vi "LSMcontroller_v64_updatedwaveformhandling.vi"() -> ()   [LabVIEW 2015] (continued)
                n4212 = call "waveformsAObuffer.vi"("command"="get") -> ("AO wf out"=w1168:waveform(dbl)[])  [unwired: 1 in]
                n4213 = local read "wavdet"() -> (w1158:bool)
                n4214 = call "waveformsDObuffer.vi"("command"="get") -> ("DO wf out"=w1164:digitalwaveform[])  [unwired: 1 in]
                n4215 = call "correctwaveformsizetemp.vi"("new sampling frequency (Hz)"=w1155, "start"=FALSE, "reference waveforms to"=w1159, "Analog waveforms in"=w1168, "stop"=FALSE, "Digital waveforms in"=w1164) -> ("analog wf out"=w1162:waveform(dbl)[], "Digital wf out"=w1160:digitalwaveform[], "measpoints"=w1157:i32)
                n4216 = local write "Analog Lines Plot"(w1162) -> ()
                n4217 = call "GetNumCamFramesv2.vi"("Digital Waveform Graph"=w1160) -> ("Numeric"=w1161:i32)  [unwired: 10 in]
                n4218 = local write "Digital Lines Plot"(w1160) -> ()
                n4219 = call "waveformsDObuffer.vi"("DO wf in"=w1160, "command"="set") -> ()  [unwired: 1 out]
                n4220 = call "waveformsAObuffer.vi"("AO wf in"=w1162, "command"="set") -> ()  [unwired: 1 out]
                n4221 = local write "Total Camera Frames"(w1161) -> ()
                n4222 = case shown="True" w1158 {
                  tunnel: w1157 -> [_ w1171]
                  frame False {
                  }
                  frame True {
                    n4223 = local write "# of frames"(w1171) -> ()
                  }
                }
              }
              frame #3 {
                n4224 = local read "finite samples"() -> (w1172:bool)
                n4225 = local read "continuous"() -> (w1173:bool)
                n4226 = local read "wavdet"() -> (w1174:bool)
                n4227 = call "2pparameters.vi"("command"="get") -> ("params out"=w1177:T10)  [unwired: 1 in]
                n4228 = Bundle By Name(cluster=w1177, "finite"=w1172, "cont"=w1173, "wavdet"=w1174) -> (w1175:T10)
                n4229 = call "2pparameters.vi"("Params in"=w1175, "command"="set") -> ()  [unwired: 1 out]
              }
            }
          }
          event "load changed AOsq": Value Change {
            n4230 = event-data() -> ("NewVal"=w1179:bool)  [unwired: 1 in, 5 out]
            n4231 = case shown="True" w1179 {
              frame False {
              }
              frame True {
                n4232 = stacked-sequence {
                  seq-local: [_ _ w1287 _ _] -> [_ _ _ w1309 _]
                  seq-local: [_ _ w1286 _ _] -> [_ _ _ w1308 _]
                  frame #0 {
                    n4233 = local read "Measurement"() -> (w1181:T4)
                    n4234 = local write "changeAOsq"(TRUE ("addAO")) -> ()
                    n4235 = case shown="\"X-Y-t movie\", Default" w1181 {
                      frame "X-Y-t movie", Default {
                        n4236 = local read "avpp"() -> (w1202:i32)
                        n4237 = local read "Angle ref"() -> (w1201:dbl)
                        n4238 = local read "ROI Type"() -> (w1200:u16)
                        n4239 = local read "xpixels ref"() -> (w1197:i32)
                        n4240 = local read "Vx-min ref"() -> (w1196:dbl)
                        n4241 = local read "Vx-max ref"() -> (w1195:dbl)
                        n4242 = local read "ypixels ref"() -> (w1193:i32)
                        n4243 = local read "Vy-min ref"() -> (w1194:dbl)
                        n4244 = local read "Vy-max ref"() -> (w1190:dbl)
                        n4245 = local read "Sampling rate"() -> (w1184:dbl)
                        n4246 = local read "finite samples"() -> (w1185:bool)
                        n4247 = local read "continuous"() -> (w1188:bool)
                        n4248 = local read "wavdet"() -> (w1189:bool)
                        n4249 = local read "# of frames"() -> (w1187:i32)
                        n4250 = local read "maxbufferAI"() -> (w1186:i32)
                        n4251 = local read "Override AI buffer"() -> (w1182:bool)
                        n4252 = call "2pparameters.vi"("command"="get") -> ("params out"=w1199:T10)  [unwired: 1 in]
                        n4253 = Bundle By Name(cluster=w1199, "type"="X-Y-t movie", "avpp"=w1202, "Angle Img"=w1201, "Xpixels Img"=w1197, "Vx-min Img"=w1196, "VX-max Img"=w1195, "Ypixels Img"=w1193, "Vy-min Img"=w1194, "Vy-max Img"=w1190, "srate"=w1184, "srate Img"=w1184, "finite"=w1185, "cont"=w1188, "wavdet"=w1189, "measpoints"=w1187, "maxbufferAI"=w1186, "Drawing Mode"=w1200, "Vz-reset"=0.0, "AIoverride"=w1182) -> (w1191:T10)
                        n4254 = call "2pparameters.vi"("Params in"=w1191, "command"="set") -> ()  [unwired: 1 out]
                      }
                      frame "X-Y-Z stack" {
                        n4255 = call "2pparameters.vi"("command"="get") -> ("params out"=w1206:T10)  [unwired: 1 in]
                        n4256 = Bundle By Name(cluster=w1206, "type"="X-Y-Z stack") -> (w1204:T10)
                        n4257 = call "2pparameters.vi"("Params in"=w1204, "command"="set") -> ()  [unwired: 1 out]
                      }
                      frame "Lifetime (scan)" {
                        n4258 = call "2pparameters.vi"("command"="get") -> ("params out"=w1211:T10)  [unwired: 1 in]
                        n4259 = Bundle By Name(cluster=w1211, "type"="Lifetime (scan)") -> (w1209:T10)
                        n4260 = call "2pparameters.vi"("Params in"=w1209, "command"="set") -> ()  [unwired: 1 out]
                      }
                      frame "Lifetime (contour)" {
                        n4261 = local read "Vy-min draw"() -> (w1221:dbl)
                        n4262 = local read "Vy-max draw"() -> (w1220:dbl)
                        n4263 = local read "Vx-min draw"() -> (w1223:dbl)
                        n4264 = local read "Vx-max draw"() -> (w1222:dbl)
                        n4265 = local read "xpixels ref"() -> (w1219:i32)
                        n4266 = local read "ypixels ref"() -> (w1218:i32)
                        n4267 = local read "ROI Type"() -> (w1217:u16)
                        n4268 = local read "srateAODOtt"() -> (w1228:dbl)
                        n4269 = local read "# of frames"() -> (w1233:i32)
                        n4270 = local read "refreshtime"() -> (w1225:dbl)
                        n4271 = local read "Pel"() -> (w1216:dbl)
                        n4272 = local read "bin"() -> (w1231:dbl)
                        n4273 = local read "Override AI buffer"() -> (w1214:bool)
                        n4274 = local read "finite samples"() -> (w1240:bool)
                        n4275 = local read "srateAODOtt"() -> (w1227:dbl)
                        n4276 = local read "srateAODOtt"() -> (w1234:dbl)
                        n4277 = local read "continuous"() -> (w1239:bool)
                        n4278 = local read "Angle ref"() -> (w1224:dbl)
                        n4279 = local read "wavdet"() -> (w1241:bool)
                        n4280 = local read "Vx-ref"() -> (w1236:dbl)
                        n4281 = local read "Vy-ref"() -> (w1238:dbl)
                        n4282 = local read "avpp"() -> (w1237:i32)
                        n4283 = call "tt_timeandsamples.vi"("bin"=w1231, "refreshtime"=w1225, "srateAODOtt"=w1228, "tot#ofsamples"=w1233) -> ("refreshrate"=w1229:dbl, "refreshbuffer"=w1230:i32, "timetracecycles"=w1235:i32)  [unwired: 5 in]
                        n4284 = local read "bin"() -> (w1232:dbl)
                        n4285 = call "2pparameters.vi"("command"="get") -> ("params out"=w1244:T10)  [unwired: 1 in]
                        n4286 = Bundle By Name(cluster=w1244, "Drawing Mode"=w1217, "measpoints"=w1233, "tt_cycles"=w1235, "refreshbuffer"=w1230, "refreshrate"=w1229, "Vx-ref"=w1236, "Vy-ref"=w1238, "srate"=w1227, "finite"=w1240, "cont"=w1239, "wavdet"=w1241, "avpp"=w1237, "srateAODO"=w1234, "bufferAI"=w1230, "bin"=w1232, "Angle Img"=w1224, "Vxminref"=w1223, "Vxmaxref"=w1222, "Vyminref"=w1221, "Vymaxref"=w1220, "Xpixels Img"=w1219, "Ypixels Img"=w1218, "Pel"=w1216, "Vz-reset"=0.0, "AIoverride"=w1214, "type"="Lifetime (contour)") -> (w1242:T10)
                        n4287 = Reciprocal(x=w1229) -> (1/x=w1226:dbl)
                        n4288 = local write "refreshtime"(w1226) -> ()
                        n4289 = call "2pparameters.vi"("Params in"=w1242, "command"="set") -> ()  [unwired: 1 out]
                      }
                      frame "X-Y-Z-t movie" {
                      }
                      frame "linescan" {
                      }
                      frame "Timetrace" {
                        n4290 = local read "Vy-min draw"() -> (w1254:dbl)
                        n4291 = local read "Vy-max draw"() -> (w1253:dbl)
                        n4292 = local read "Vx-min draw"() -> (w1256:dbl)
                        n4293 = local read "Vx-max draw"() -> (w1255:dbl)
                        n4294 = local read "xpixels ref"() -> (w1252:i32)
                        n4295 = local read "ypixels ref"() -> (w1251:i32)
                        n4296 = local read "ROI Type"() -> (w1250:u16)
                        n4297 = local read "srateAODOtt"() -> (w1261:dbl)
                        n4298 = local read "# of frames"() -> (w1266:i32)
                        n4299 = local read "refreshtime"() -> (w1258:dbl)
                        n4300 = local read "Pel"() -> (w1249:dbl)
                        n4301 = local read "bin"() -> (w1264:dbl)
                        n4302 = local read "Override AI buffer"() -> (w1247:bool)
                        n4303 = local read "finite samples"() -> (w1273:bool)
                        n4304 = local read "srateAODOtt"() -> (w1260:dbl)
                        n4305 = local read "srateAODOtt"() -> (w1267:dbl)
                        n4306 = local read "continuous"() -> (w1272:bool)
                        n4307 = local read "Angle ref"() -> (w1257:dbl)
                        n4308 = local read "wavdet"() -> (w1274:bool)
                        n4309 = local read "Vx-ref"() -> (w1269:dbl)
                        n4310 = local read "Vy-ref"() -> (w1271:dbl)
                        n4311 = local read "avpp"() -> (w1270:i32)
                        n4312 = call "tt_timeandsamples.vi"("bin"=w1264, "refreshtime"=w1258, "srateAODOtt"=w1261, "tot#ofsamples"=w1266) -> ("refreshrate"=w1262:dbl, "refreshbuffer"=w1263:i32, "timetracecycles"=w1268:i32)  [unwired: 5 in]
                        n4313 = local read "bin"() -> (w1265:dbl)
                        n4314 = call "2pparameters.vi"("command"="get") -> ("params out"=w1277:T10)  [unwired: 1 in]
                        n4315 = Bundle By Name(cluster=w1277, "Drawing Mode"=w1250, "measpoints"=w1266, "tt_cycles"=w1268, "refreshbuffer"=w1263, "refreshrate"=w1262, "Vx-ref"=w1269, "Vy-ref"=w1271, "srate"=w1260, "finite"=w1273, "cont"=w1272, "wavdet"=w1274, "avpp"=w1270, "srateAODO"=w1267, "bufferAI"=w1263, "bin"=w1265, "Angle Img"=w1257, "Vxminref"=w1256, "Vxmaxref"=w1255, "Vyminref"=w1254, "Vymaxref"=w1253, "Xpixels Img"=w1252, "Ypixels Img"=w1251, "Pel"=w1249, "Vz-reset"=0.0, "AIoverride"=w1247, "type"="Timetrace") -> (w1275:T10)
                        n4316 = Reciprocal(x=w1262) -> (1/x=w1259:dbl)
                        n4317 = local write "refreshtime"(w1259) -> ()
                        n4318 = call "2pparameters.vi"("Params in"=w1275, "command"="set") -> ()  [unwired: 1 out]
                      }
                      frame "Lifetime (point)" {
                      }
                    }
                  }
                  frame #1 {
                    w1280 = FALSE ("wavdet")
                    n4319 = call "2pparameters.vi"("command"="get") -> ("params out"=w1284:T10)  [unwired: 1 in]
                    n4320 = Bundle By Name(cluster=w1284, "finite"=w1280, "cont"=w1280, "wavdet"=TRUE) -> (w1281:T10)
                    n4321 = call "2pparameters.vi"("Params in"=w1281, "command"="set") -> ()  [unwired: 1 out]
                  }
                  frame #2 {
                    n4322 = local read "AO channels"() -> (w1289:u32)
                    n4323 = call "2pparameters.vi"("command"="get") -> ("params out"=w1291:T10)  [unwired: 1 in]
                    n4324 = Unbundle By Name(w1291) -> ("aAO"=w1290:u32[])
                    n4325 = Search 1D Array(1D array=w1290, element=w1289) -> (index of element=w1287:i32)  [unwired: 1 in]
                    n4326 = Greater?(x=w1287, y=-1) -> (0:w1286:bool)
                    n4327 = case shown="True" w1286 {
                      tunnel: w1287 -> [_ w1305]
                      frame False {
                      }
                      frame True {
                        n4328 = local read "Meastab"() -> (w1294:enum32{"X-Y Image", "Linescan", "Timetrace"})
                        n4329 = case shown="\"Timetrace\"" w1294 {
                          tunnel: [w1306 w1307] -> w1293
                          frame "X-Y Image", Default {
                            n4330 = local read "Sampling rate"() -> (w1306:dbl)
                          }
                          frame "Timetrace" {
                            n4331 = local read "srateAODOtt"() -> (w1307:dbl)
                          }
                        }
                        n4332 = local read "Start amplitude (V)"() -> (w1302:dbl)
                        n4333 = local read "phase shift (ms)"() -> (w1297:dbl)
                        n4334 = local read "Step size (V)"() -> (w1300:dbl)
                        n4335 = local read "Baseline (V)"() -> (w1301:dbl)
                        n4336 = local read "Period (ms)"() -> (w1298:dbl)
                        n4337 = local read "padding value"() -> (w1295:dbl)
                        n4338 = local read "Repeats"() -> (w1304:dbl)
                        n4339 = local read "Cycles"() -> (w1303:dbl)
                        n4340 = local read "DC (%)"() -> (w1299:dbl)
                        n4341 = local read "Pulses"() -> (w1296:dbl)
                        n4342 = call "replace AO square wf param.vi"("Baseline (V)"=w1301, "Start amplitude (V)"=w1302, "Cycles"=w1303, "Repeats"=w1304, "index of AO wave"=w1305, "Step size (V)"=w1300, "DC (%)"=w1299, "Sampling frequency (Hz)"=w1293, "Period (ms)"=w1298, "Cycle length (s)"=w1297, "Pulses"=w1296, "padding value"=w1295) -> ()  [unwired: 4 in]
                      }
                    }
                  }
                  frame #3 {
                    n4343 = case shown="True" w1308 {
                      tunnel: w1309 -> [_ w1317]
                      frame False {
                      }
                      frame True {
                        n4344 = call "waveformparamsv2.vi"("command"="get") -> ("Params out"=w1331:T14)  [unwired: 4 in, 2 out]
                        n4345 = Unbundle By Name(w1331) -> ("AO parameters"=w1330:T15)
                        n4346 = local read "Meastab"() -> (w1312:enum32{"X-Y Image", "Linescan", "Timetrace"})
                        n4347 = case shown="\"Timetrace\"" w1312 {
                          tunnel: [w1333 w1334] -> w1321
                          frame "X-Y Image", Default {
                            n4348 = local read "Sampling rate"() -> (w1333:dbl)
                          }
                          frame "Timetrace" {
                            n4349 = local read "srateAODOtt"() -> (w1334:dbl)
                          }
                        }
                        n4350 = Index Array(array=w1330, index=w1317) -> (element=w1319:T16)
                        n4351 = call "waveformsAObuffer.vi"("command"="get") -> ("AO wf out"=w1318:waveform(dbl)[])  [unwired: 1 in]
                        n4352 = call "generateRampedSquareWave_fromAOparameters.vi"("AO params"=w1319) -> ("Waveform"=w1316:waveform(dbl))  [unwired: 1 out]
                        n4353 = property on="refwf" class="Ring (strict)"() -> ("RingText.Text"=w1320:string)  [unwired: 2 in, 2 out]
                        n4354 = Replace Array Subset(array=w1318, new element=w1316, index=w1317) -> (w1315:waveform(dbl)[])
                        n4355 = call "waveformsDObuffer.vi"("command"="get") -> ("DO wf out"=w1326:digitalwaveform[])  [unwired: 1 in]
                        n4356 = call "correctwaveformsizetemp.vi"("new sampling frequency (Hz)"=w1321, "start"=FALSE, "reference waveforms to"=w1320, "Analog waveforms in"=w1315, "stop"=FALSE, "Digital waveforms in"=w1326) -> ("analog wf out"=w1324:waveform(dbl)[], "Digital wf out"=w1322:digitalwaveform[], "measpoints"=w1313:i32)
                        n4357 = local read "wavdet"() -> (w1314:bool)
                        n4358 = local write "Analog Lines Plot"(w1324) -> ()
                        n4359 = call "GetNumCamFramesv2.vi"("Digital Waveform Graph"=w1322) -> ("Numeric"=w1323:i32)  [unwired: 10 in]
                        n4360 = local write "Digital Lines Plot"(w1322) -> ()
                        n4361 = call "waveformsAObuffer.vi"("AO wf in"=w1324, "command"="set") -> ()  [unwired: 1 out]
                        n4362 = call "waveformsDObuffer.vi"("DO wf in"=w1322, "command"="set") -> ()  [unwired: 1 out]
                        n4363 = local write "Total Camera Frames"(w1323) -> ()
                        n4364 = case shown="True" w1314 {
                          tunnel: w1313 -> [_ w1335]
                          frame False {
                          }
                          frame True {
                            n4365 = local write "# of frames"(w1335) -> ()
                          }
                        }
                      }
                    }
                  }
                  frame #4 {
                    w1337 = FALSE ("addAO")
                    n4366 = local read "finite samples"() -> (w1338:bool)
                    n4367 = local read "continuous"() -> (w1339:bool)
                    n4368 = local read "wavdet"() -> (w1340:bool)
                    n4369 = local write "changeAOsq"(w1337) -> ()
                    n4370 = property on="load changed AOsq" class="Bool (strict)"("Val(Sgnl)"=w1337) -> ()  [unwired: 2 in, 2 out]
                    n4371 = call "2pparameters.vi"("command"="get") -> ("params out"=w1343:T10)  [unwired: 1 in]
                    n4372 = Bundle By Name(cluster=w1343, "finite"=w1338, "cont"=w1339, "wavdet"=w1340) -> (w1341:T10)
                    n4373 = local write "not loaded"(FALSE ("not loaded")) -> ()
                    n4374 = call "2pparameters.vi"("Params in"=w1341, "command"="set") -> ()  [unwired: 1 out]
                  }
                }
              }
            }
          }
          event "load changed AOtri": Value Change {
            n4375 = event-data() -> ("NewVal"=w1345:bool)  [unwired: 1 in, 5 out]
            n4376 = case shown="True" w1345 {
              frame False {
              }
              frame True {
                n4377 = stacked-sequence {
                  seq-local: [_ _ w1453 _ _] -> [_ _ _ w1471 _]
                  seq-local: [_ _ w1452 _ _] -> [_ _ _ w1470 _]
                  frame #0 {
                    n4378 = local read "Measurement"() -> (w1347:T4)
                    n4379 = local write "changeAOtri"(TRUE ("addAO")) -> ()
                    n4380 = case shown="\"X-Y-t movie\", Default" w1347 {
                      frame "X-Y-t movie", Default {
                        n4381 = local read "avpp"() -> (w1368:i32)
                        n4382 = local read "Angle ref"() -> (w1367:dbl)
                        n4383 = local read "ROI Type"() -> (w1366:u16)
                        n4384 = local read "xpixels ref"() -> (w1363:i32)
                        n4385 = local read "Vx-min ref"() -> (w1362:dbl)
                        n4386 = local read "Vx-max ref"() -> (w1361:dbl)
                        n4387 = local read "ypixels ref"() -> (w1359:i32)
                        n4388 = local read "Vy-min ref"() -> (w1360:dbl)
                        n4389 = local read "Vy-max ref"() -> (w1356:dbl)
                        n4390 = local read "Sampling rate"() -> (w1350:dbl)
                        n4391 = local read "finite samples"() -> (w1351:bool)
                        n4392 = local read "continuous"() -> (w1354:bool)
                        n4393 = local read "wavdet"() -> (w1355:bool)
                        n4394 = local read "# of frames"() -> (w1353:i32)
                        n4395 = local read "maxbufferAI"() -> (w1352:i32)
                        n4396 = local read "Override AI buffer"() -> (w1348:bool)
                        n4397 = call "2pparameters.vi"("command"="get") -> ("params out"=w1365:T10)  [unwired: 1 in]
                        n4398 = Bundle By Name(cluster=w1365, "type"="X-Y-t movie", "avpp"=w1368, "Angle Img"=w1367, "Xpixels Img"=w1363, "Vx-min Img"=w1362, "VX-max Img"=w1361, "Ypixels Img"=w1359, "Vy-min Img"=w1360, "Vy-max Img"=w1356, "srate"=w1350, "srate Img"=w1350, "finite"=w1351, "cont"=w1354, "wavdet"=w1355, "measpoints"=w1353, "maxbufferAI"=w1352, "Drawing Mode"=w1366, "Vz-reset"=0.0, "AIoverride"=w1348) -> (w1357:T10)
                        n4399 = call "2pparameters.vi"("Params in"=w1357, "command"="set") -> ()  [unwired: 1 out]
                      }
                      frame "X-Y-Z stack" {
                        n4400 = call "2pparameters.vi"("command"="get") -> ("params out"=w1372:T10)  [unwired: 1 in]
                        n4401 = Bundle By Name(cluster=w1372, "type"="X-Y-Z stack") -> (w1370:T10)
                        n4402 = call "2pparameters.vi"("Params in"=w1370, "command"="set") -> ()  [unwired: 1 out]
                      }
                      frame "Lifetime (scan)" {
                        n4403 = call "2pparameters.vi"("command"="get") -> ("params out"=w1377:T10)  [unwired: 1 in]
                        n4404 = Bundle By Name(cluster=w1377, "type"="Lifetime (scan)") -> (w1375:T10)
                        n4405 = call "2pparameters.vi"("Params in"=w1375, "command"="set") -> ()  [unwired: 1 out]
                      }
                      frame "Lifetime (contour)" {
                        n4406 = local read "Vy-min draw"() -> (w1387:dbl)
                        n4407 = local read "Vy-max draw"() -> (w1386:dbl)
                        n4408 = local read "Vx-min draw"() -> (w1389:dbl)
                        n4409 = local read "Vx-max draw"() -> (w1388:dbl)
                        n4410 = local read "xpixels ref"() -> (w1385:i32)
                        n4411 = local read "ypixels ref"() -> (w1384:i32)
                        n4412 = local read "ROI Type"() -> (w1383:u16)
                        n4413 = local read "srateAODOtt"() -> (w1394:dbl)
                        n4414 = local read "# of frames"() -> (w1399:i32)
                        n4415 = local read "refreshtime"() -> (w1391:dbl)
                        n4416 = local read "Pel"() -> (w1382:dbl)
                        n4417 = local read "bin"() -> (w1397:dbl)
                        n4418 = local read "Override AI buffer"() -> (w1380:bool)
                        n4419 = local read "finite samples"() -> (w1406:bool)
                        n4420 = local read "srateAODOtt"() -> (w1393:dbl)
                        n4421 = local read "srateAODOtt"() -> (w1400:dbl)
                        n4422 = local read "continuous"() -> (w1405:bool)
                        n4423 = local read "Angle ref"() -> (w1390:dbl)
                        n4424 = local read "wavdet"() -> (w1407:bool)
                        n4425 = local read "Vx-ref"() -> (w1402:dbl)
                        n4426 = local read "Vy-ref"() -> (w1404:dbl)
                        n4427 = local read "avpp"() -> (w1403:i32)
                        n4428 = call "tt_timeandsamples.vi"("bin"=w1397, "refreshtime"=w1391, "srateAODOtt"=w1394, "tot#ofsamples"=w1399) -> ("refreshrate"=w1395:dbl, "refreshbuffer"=w1396:i32, "timetracecycles"=w1401:i32)  [unwired: 5 in]
                        n4429 = local read "bin"() -> (w1398:dbl)
                        n4430 = call "2pparameters.vi"("command"="get") -> ("params out"=w1410:T10)  [unwired: 1 in]
                        n4431 = Bundle By Name(cluster=w1410, "Drawing Mode"=w1383, "measpoints"=w1399, "tt_cycles"=w1401, "refreshbuffer"=w1396, "refreshrate"=w1395, "Vx-ref"=w1402, "Vy-ref"=w1404, "srate"=w1393, "finite"=w1406, "cont"=w1405, "wavdet"=w1407, "avpp"=w1403, "srateAODO"=w1400, "bufferAI"=w1396, "bin"=w1398, "Angle Img"=w1390, "Vxminref"=w1389, "Vxmaxref"=w1388, "Vyminref"=w1387, "Vymaxref"=w1386, "Xpixels Img"=w1385, "Ypixels Img"=w1384, "Pel"=w1382, "Vz-reset"=0.0, "AIoverride"=w1380, "type"="Lifetime (contour)") -> (w1408:T10)
                        n4432 = Reciprocal(x=w1395) -> (1/x=w1392:dbl)
                        n4433 = local write "refreshtime"(w1392) -> ()
                        n4434 = call "2pparameters.vi"("Params in"=w1408, "command"="set") -> ()  [unwired: 1 out]
                      }
                      frame "X-Y-Z-t movie" {
                      }
                      frame "linescan" {
                      }
                      frame "Timetrace" {
                        n4435 = local read "Vy-min draw"() -> (w1420:dbl)
                        n4436 = local read "Vy-max draw"() -> (w1419:dbl)
                        n4437 = local read "Vx-min draw"() -> (w1422:dbl)
                        n4438 = local read "Vx-max draw"() -> (w1421:dbl)
                        n4439 = local read "xpixels ref"() -> (w1418:i32)
                        n4440 = local read "ypixels ref"() -> (w1417:i32)
                        n4441 = local read "ROI Type"() -> (w1416:u16)
                        n4442 = local read "srateAODOtt"() -> (w1427:dbl)
                        n4443 = local read "# of frames"() -> (w1432:i32)
                        n4444 = local read "refreshtime"() -> (w1424:dbl)
                        n4445 = local read "Pel"() -> (w1415:dbl)
                        n4446 = local read "bin"() -> (w1430:dbl)
                        n4447 = local read "Override AI buffer"() -> (w1413:bool)
                        n4448 = local read "finite samples"() -> (w1439:bool)
                        n4449 = local read "srateAODOtt"() -> (w1426:dbl)
                        n4450 = local read "srateAODOtt"() -> (w1433:dbl)
                        n4451 = local read "continuous"() -> (w1438:bool)
                        n4452 = local read "Angle ref"() -> (w1423:dbl)
                        n4453 = local read "wavdet"() -> (w1440:bool)
                        n4454 = local read "Vx-ref"() -> (w1435:dbl)
                        n4455 = local read "Vy-ref"() -> (w1437:dbl)
                        n4456 = local read "avpp"() -> (w1436:i32)
                        n4457 = call "tt_timeandsamples.vi"("bin"=w1430, "refreshtime"=w1424, "srateAODOtt"=w1427, "tot#ofsamples"=w1432) -> ("refreshrate"=w1428:dbl, "refreshbuffer"=w1429:i32, "timetracecycles"=w1434:i32)  [unwired: 5 in]
                        n4458 = local read "bin"() -> (w1431:dbl)
                        n4459 = call "2pparameters.vi"("command"="get") -> ("params out"=w1443:T10)  [unwired: 1 in]
                        n4460 = Bundle By Name(cluster=w1443, "Drawing Mode"=w1416, "measpoints"=w1432, "tt_cycles"=w1434, "refreshbuffer"=w1429, "refreshrate"=w1428, "Vx-ref"=w1435, "Vy-ref"=w1437, "srate"=w1426, "finite"=w1439, "cont"=w1438, "wavdet"=w1440, "avpp"=w1436, "srateAODO"=w1433, "bufferAI"=w1429, "bin"=w1431, "Angle Img"=w1423, "Vxminref"=w1422, "Vxmaxref"=w1421, "Vyminref"=w1420, "Vymaxref"=w1419, "Xpixels Img"=w1418, "Ypixels Img"=w1417, "Pel"=w1415, "Vz-reset"=0.0, "AIoverride"=w1413, "type"="Timetrace") -> (w1441:T10)
                        n4461 = Reciprocal(x=w1428) -> (1/x=w1425:dbl)
                        n4462 = local write "refreshtime"(w1425) -> ()
                        n4463 = call "2pparameters.vi"("Params in"=w1441, "command"="set") -> ()  [unwired: 1 out]
                      }
                      frame "Lifetime (point)" {
                      }
                    }
                  }
                  frame #1 {
                    w1446 = FALSE ("wavdet")
                    n4464 = call "2pparameters.vi"("command"="get") -> ("params out"=w1450:T10)  [unwired: 1 in]
                    n4465 = Bundle By Name(cluster=w1450, "finite"=w1446, "cont"=w1446, "wavdet"=TRUE) -> (w1447:T10)
                    n4466 = call "2pparameters.vi"("Params in"=w1447, "command"="set") -> ()  [unwired: 1 out]
                  }
                  frame #2 {
                    n4467 = local read "AO channels"() -> (w1455:u32)
                    n4468 = call "2pparameters.vi"("command"="get") -> ("params out"=w1457:T10)  [unwired: 1 in]
                    n4469 = Unbundle By Name(w1457) -> ("aAO"=w1456:u32[])
                    n4470 = Search 1D Array(1D array=w1456, element=w1455) -> (index of element=w1453:i32)  [unwired: 1 in]
                    n4471 = Greater?(x=w1453, y=-1) -> (0:w1452:bool)
                    n4472 = case shown="True" w1452 {
                      tunnel: w1453 -> [_ w1467]
                      frame False {
                      }
                      frame True {
                        n4473 = local read "Meastab"() -> (w1460:enum32{"X-Y Image", "Linescan", "Timetrace"})
                        n4474 = local read "Tri padding value"() -> (w1461:dbl)
                        n4475 = local read "Amplitude (V)"() -> (w1465:dbl)
                        n4476 = local read "Tri Phase (s)"() -> (w1462:dbl)
                        n4477 = local read "Tri Repeats"() -> (w1463:dbl)
                        n4478 = local read "Frequency"() -> (w1464:dbl)
                        n4479 = local read "Offset (V)"() -> (w1466:dbl)
                        n4480 = case shown="\"Timetrace\"" w1460 {
                          tunnel: [w1468 w1469] -> w1459
                          frame "X-Y Image", Default {
                            n4481 = local read "Sampling rate"() -> (w1468:dbl)
                          }
                          frame "Timetrace" {
                            n4482 = local read "srateAODOtt"() -> (w1469:dbl)
                          }
                        }
                        n4483 = call "replace AO tri wf param.vi"("padding value"=w1461, "index of AO wave"=w1467, "Tri phase"=w1462, "Sampling frequency (Hz)"=w1459, "Tri Repeats"=w1463, "Frequency"=w1464, "Amplitude (V)"=w1465, "Offset (V)"=w1466) -> ()
                      }
                    }
                  }
                  frame #3 {
                    n4484 = case shown="True" w1470 {
                      tunnel: w1471 -> [_ w1480]
                      frame False {
                      }
                      frame True {
                        n4485 = call "waveformparamsv2.vi"("command"="get") -> ("Params out"=w1493:T14)  [unwired: 4 in, 2 out]
                        n4486 = Unbundle By Name(w1493) -> ("AO parameters"=w1492:T15)
                        n4487 = local read "Meastab"() -> (w1475:enum32{"X-Y Image", "Linescan", "Timetrace"})
                        n4488 = case shown="\"Timetrace\"" w1475 {
                          tunnel: [w1495 w1496] -> w1474
                          frame "X-Y Image", Default {
                            n4489 = local read "Sampling rate"() -> (w1495:dbl)
                          }
                          frame "Timetrace" {
                            n4490 = local read "srateAODOtt"() -> (w1496:dbl)
                          }
                        }
                        n4491 = Index Array(array=w1492, index=w1480) -> (element=w1482:T16)
                        n4492 = call "waveformsAObuffer.vi"("command"="get") -> ("AO wf out"=w1481:waveform(dbl)[])  [unwired: 1 in]
                        n4493 = call "generateTriWave_fromAOparameters.vi"("AO params"=w1482) -> ("Waveform"=w1479:waveform(dbl))  [unwired: 1 out]
                        n4494 = property on="refwf" class="Ring (strict)"() -> ("RingText.Text"=w1483:string)  [unwired: 2 in, 2 out]
                        n4495 = Replace Array Subset(array=w1481, new element=w1479, index=w1480) -> (w1478:waveform(dbl)[])
                        n4496 = call "waveformsDObuffer.vi"("command"="get") -> ("DO wf out"=w1488:digitalwaveform[])  [unwired: 1 in]
                        n4497 = call "correctwaveformsizetemp.vi"("new sampling frequency (Hz)"=w1474, "start"=FALSE, "reference waveforms to"=w1483, "Analog waveforms in"=w1478, "stop"=FALSE, "Digital waveforms in"=w1488) -> ("analog wf out"=w1486:waveform(dbl)[], "Digital wf out"=w1484:digitalwaveform[], "measpoints"=w1476:i32)
                        n4498 = local read "wavdet"() -> (w1477:bool)
                        n4499 = local write "Analog Lines Plot"(w1486) -> ()
                        n4500 = call "GetNumCamFramesv2.vi"("Digital Waveform Graph"=w1484) -> ("Numeric"=w1485:i32)  [unwired: 10 in]
                        n4501 = local write "Digital Lines Plot"(w1484) -> ()
                        n4502 = call "waveformsAObuffer.vi"("AO wf in"=w1486, "command"="set") -> ()  [unwired: 1 out]
                        n4503 = call "waveformsDObuffer.vi"("DO wf in"=w1484, "command"="set") -> ()  [unwired: 1 out]
                        n4504 = local write "Total Camera Frames"(w1485) -> ()
                        n4505 = case shown="True" w1477 {
                          tunnel: w1476 -> [_ w1497]
                          frame False {
                          }
                          frame True {
                            n4506 = local write "# of frames"(w1497) -> ()
                          }
                        }
                      }
                    }
                  }
                  frame #4 {
                    w1499 = FALSE ("addAO")
                    n4507 = local write "not loadedtri"(FALSE ("not loadedtri")) -> ()
                    n4508 = local write "changeAOtri"(w1499) -> ()
                    n4509 = property on="load changed AOtri" class="Bool (strict)"("Val(Sgnl)"=w1499) -> ()  [unwired: 2 in, 2 out]
                    n4510 = local read "finite samples"() -> (w1500:bool)
                    n4511 = local read "continuous"() -> (w1501:bool)
                    n4512 = local read "wavdet"() -> (w1502:bool)
                    n4513 = call "2pparameters.vi"("command"="get") -> ("params out"=w1505:T10)  [unwired: 1 in]
                    n4514 = Bundle By Name(cluster=w1505, "finite"=w1500, "cont"=w1501, "wavdet"=w1502) -> (w1503:T10)
                    n4515 = call "2pparameters.vi"("Params in"=w1503, "command"="set") -> ()  [unwired: 1 out]
                  }
                }
              }
            }
          }
          event "Load Matlab Waveform": Value Change {
            n4516 = event-data() -> ("NewVal"=w1507:bool)  [unwired: 1 in, 5 out]
            n4517 = case shown="True" w1507 {
              frame False {
              }
              frame True {
                n4518 = stacked-sequence {
                  seq-local: [_ _ w1615 _ _] -> [_ _ _ w1630 _]
                  seq-local: [_ _ w1614 _ _] -> [_ _ _ w1629 _]
                  frame #0 {
                    n4519 = local read "Measurement"() -> (w1509:T4)
                    n4520 = case shown="\"X-Y-t movie\", Default" w1509 {
                      frame "X-Y-t movie", Default {
                        n4521 = local read "avpp"() -> (w1530:i32)
                        n4522 = local read "Angle ref"() -> (w1529:dbl)
                        n4523 = local read "ROI Type"() -> (w1528:u16)
                        n4524 = local read "xpixels ref"() -> (w1525:i32)
                        n4525 = local read "Vx-min ref"() -> (w1524:dbl)
                        n4526 = local read "Vx-max ref"() -> (w1523:dbl)
                        n4527 = local read "ypixels ref"() -> (w1521:i32)
                        n4528 = local read "Vy-min ref"() -> (w1522:dbl)
                        n4529 = local read "Vy-max ref"() -> (w1518:dbl)
                        n4530 = local read "Sampling rate"() -> (w1512:dbl)
                        n4531 = local read "finite samples"() -> (w1513:bool)
                        n4532 = local read "continuous"() -> (w1516:bool)
                        n4533 = local read "wavdet"() -> (w1517:bool)
                        n4534 = local read "# of frames"() -> (w1515:i32)
                        n4535 = local read "maxbufferAI"() -> (w1514:i32)
                        n4536 = local read "Override AI buffer"() -> (w1510:bool)
                        n4537 = call "2pparameters.vi"("command"="get") -> ("params out"=w1527:T10)  [unwired: 1 in]
                        n4538 = Bundle By Name(cluster=w1527, "type"="X-Y-t movie", "avpp"=w1530, "Angle Img"=w1529, "Xpixels Img"=w1525, "Vx-min Img"=w1524, "VX-max Img"=w1523, "Ypixels Img"=w1521, "Vy-min Img"=w1522, "Vy-max Img"=w1518, "srate"=w1512, "srate Img"=w1512, "finite"=w1513, "cont"=w1516, "wavdet"=w1517, "measpoints"=w1515, "maxbufferAI"=w1514, "Drawing Mode"=w1528, "Vz-reset"=0.0, "AIoverride"=w1510) -> (w1519:T10)
                        n4539 = call "2pparameters.vi"("Params in"=w1519, "command"="set") -> ()  [unwired: 1 out]
                      }
                      frame "X-Y-Z stack" {
                        n4540 = call "2pparameters.vi"("command"="get") -> ("params out"=w1534:T10)  [unwired: 1 in]
                        n4541 = Bundle By Name(cluster=w1534, "type"="X-Y-Z stack") -> (w1532:T10)
                        n4542 = call "2pparameters.vi"("Params in"=w1532, "command"="set") -> ()  [unwired: 1 out]
                      }
                      frame "Lifetime (scan)" {
                        n4543 = call "2pparameters.vi"("command"="get") -> ("params out"=w1539:T10)  [unwired: 1 in]
                        n4544 = Bundle By Name(cluster=w1539, "type"="Lifetime (scan)") -> (w1537:T10)
                        n4545 = call "2pparameters.vi"("Params in"=w1537, "command"="set") -> ()  [unwired: 1 out]
                      }
                      frame "Lifetime (contour)" {
                        n4546 = local read "Vy-min draw"() -> (w1549:dbl)
                        n4547 = local read "Vy-max draw"() -> (w1548:dbl)
                        n4548 = local read "Vx-min draw"() -> (w1551:dbl)
                        n4549 = local read "Vx-max draw"() -> (w1550:dbl)
                        n4550 = local read "xpixels ref"() -> (w1547:i32)
                        n4551 = local read "ypixels ref"() -> (w1546:i32)
                        n4552 = local read "ROI Type"() -> (w1545:u16)
                        n4553 = local read "srateAODOtt"() -> (w1556:dbl)
                        n4554 = local read "# of frames"() -> (w1561:i32)
                        n4555 = local read "refreshtime"() -> (w1553:dbl)
                        n4556 = local read "Pel"() -> (w1544:dbl)
                        n4557 = local read "bin"() -> (w1559:dbl)
                        n4558 = local read "Override AI buffer"() -> (w1542:bool)
                        n4559 = local read "finite samples"() -> (w1568:bool)
                        n4560 = local read "srateAODOtt"() -> (w1555:dbl)
                        n4561 = local read "srateAODOtt"() -> (w1562:dbl)
                        n4562 = local read "continuous"() -> (w1567:bool)
                        n4563 = local read "Angle ref"() -> (w1552:dbl)
                        n4564 = local read "wavdet"() -> (w1569:bool)
                        n4565 = local read "Vx-ref"() -> (w1564:dbl)
                        n4566 = local read "Vy-ref"() -> (w1566:dbl)
                        n4567 = local read "avpp"() -> (w1565:i32)
                        n4568 = call "tt_timeandsamples.vi"("bin"=w1559, "refreshtime"=w1553, "srateAODOtt"=w1556, "tot#ofsamples"=w1561) -> ("refreshrate"=w1557:dbl, "refreshbuffer"=w1558:i32, "timetracecycles"=w1563:i32)  [unwired: 5 in]
                        n4569 = local read "bin"() -> (w1560:dbl)
                        n4570 = call "2pparameters.vi"("command"="get") -> ("params out"=w1572:T10)  [unwired: 1 in]
                        n4571 = Bundle By Name(cluster=w1572, "Drawing Mode"=w1545, "measpoints"=w1561, "tt_cycles"=w1563, "refreshbuffer"=w1558, "refreshrate"=w1557, "Vx-ref"=w1564, "Vy-ref"=w1566, "srate"=w1555, "finite"=w1568, "cont"=w1567, "wavdet"=w1569, "avpp"=w1565, "srateAODO"=w1562, "bufferAI"=w1558, "bin"=w1560, "Angle Img"=w1552, "Vxminref"=w1551, "Vxmaxref"=w1550, "Vyminref"=w1549, "Vymaxref"=w1548, "Xpixels Img"=w1547, "Ypixels Img"=w1546, "Pel"=w1544, "Vz-reset"=0.0, "AIoverride"=w1542, "type"="Lifetime (contour)") -> (w1570:T10)
                        n4572 = Reciprocal(x=w1557) -> (1/x=w1554:dbl)
                        n4573 = local write "refreshtime"(w1554) -> ()
                        n4574 = call "2pparameters.vi"("Params in"=w1570, "command"="set") -> ()  [unwired: 1 out]
                      }
                      frame "X-Y-Z-t movie" {
                      }
                      frame "linescan" {
                      }
                      frame "Timetrace" {
                        n4575 = local read "Vy-min draw"() -> (w1582:dbl)
                        n4576 = local read "Vy-max draw"() -> (w1581:dbl)
                        n4577 = local read "Vx-min draw"() -> (w1584:dbl)
                        n4578 = local read "Vx-max draw"() -> (w1583:dbl)
                        n4579 = local read "xpixels ref"() -> (w1580:i32)
                        n4580 = local read "ypixels ref"() -> (w1579:i32)
                        n4581 = local read "ROI Type"() -> (w1578:u16)
                        n4582 = local read "srateAODOtt"() -> (w1589:dbl)
                        n4583 = local read "# of frames"() -> (w1594:i32)
                        n4584 = local read "refreshtime"() -> (w1586:dbl)
                        n4585 = local read "Pel"() -> (w1577:dbl)
                        n4586 = local read "bin"() -> (w1592:dbl)
                        n4587 = local read "Override AI buffer"() -> (w1575:bool)
                        n4588 = local read "finite samples"() -> (w1601:bool)
                        n4589 = local read "srateAODOtt"() -> (w1588:dbl)
                        n4590 = local read "srateAODOtt"() -> (w1595:dbl)
                        n4591 = local read "continuous"() -> (w1600:bool)
                        n4592 = local read "Angle ref"() -> (w1585:dbl)
                        n4593 = local read "wavdet"() -> (w1602:bool)
                        n4594 = local read "Vx-ref"() -> (w1597:dbl)
                        n4595 = local read "Vy-ref"() -> (w1599:dbl)
                        n4596 = local read "avpp"() -> (w1598:i32)
                        n4597 = call "tt_timeandsamples.vi"("bin"=w1592, "refreshtime"=w1586, "srateAODOtt"=w1589, "tot#ofsamples"=w1594) -> ("refreshrate"=w1590:dbl, "refreshbuffer"=w1591:i32, "timetracecycles"=w1596:i32)  [unwired: 5 in]
                        n4598 = local read "bin"() -> (w1593:dbl)
                        n4599 = call "2pparameters.vi"("command"="get") -> ("params out"=w1605:T10)  [unwired: 1 in]
                        n4600 = Bundle By Name(cluster=w1605, "Drawing Mode"=w1578, "measpoints"=w1594, "tt_cycles"=w1596, "refreshbuffer"=w1591, "refreshrate"=w1590, "Vx-ref"=w1597, "Vy-ref"=w1599, "srate"=w1588, "finite"=w1601, "cont"=w1600, "wavdet"=w1602, "avpp"=w1598, "srateAODO"=w1595, "bufferAI"=w1591, "bin"=w1593, "Angle Img"=w1585, "Vxminref"=w1584, "Vxmaxref"=w1583, "Vyminref"=w1582, "Vymaxref"=w1581, "Xpixels Img"=w1580, "Ypixels Img"=w1579, "Pel"=w1577, "Vz-reset"=0.0, "AIoverride"=w1575, "type"="Timetrace") -> (w1603:T10)
                        n4601 = Reciprocal(x=w1590) -> (1/x=w1587:dbl)
                        n4602 = local write "refreshtime"(w1587) -> ()
                        n4603 = call "2pparameters.vi"("Params in"=w1603, "command"="set") -> ()  [unwired: 1 out]
                      }
                      frame "Lifetime (point)" {
                      }
                    }
                    n4604 = local write "changeAOmatlab"(TRUE ("addAO")) -> ()
                  }
                  frame #1 {
                    w1608 = FALSE ("wavdet")
                    n4605 = call "2pparameters.vi"("command"="get") -> ("params out"=w1612:T10)  [unwired: 1 in]
                    n4606 = Bundle By Name(cluster=w1612, "finite"=w1608, "cont"=w1608, "wavdet"=TRUE) -> (w1609:T10)
                    n4607 = call "2pparameters.vi"("Params in"=w1609, "command"="set") -> ()  [unwired: 1 out]
                  }
                  frame #2 {
                    n4608 = local read "AO channels"() -> (w1617:u32)
                    n4609 = call "2pparameters.vi"("command"="get") -> ("params out"=w1619:T10)  [unwired: 1 in]
                    n4610 = Unbundle By Name(w1619) -> ("aAO"=w1618:u32[])
                    n4611 = Search 1D Array(1D array=w1618, element=w1617) -> (index of element=w1615:i32)  [unwired: 1 in]
                    n4612 = Greater?(x=w1615, y=-1) -> (0:w1614:bool)
                    n4613 = case shown="True" w1614 {
                      tunnel: w1615 -> [_ w1626]
                      frame False {
                      }
                      frame True {
                        n4614 = local read "Meastab"() -> (w1622:enum32{"X-Y Image", "Linescan", "Timetrace"})
                        n4615 = local read "Matlab waveform path"() -> (w1624:path)
                        n4616 = local read "Matlab padding value"() -> (w1625:dbl)
                        n4617 = case shown="\"Timetrace\"" w1622 {
                          tunnel: [w1627 w1628] -> w1621
                          frame "X-Y Image", Default {
                            n4618 = local read "Sampling rate"() -> (w1627:dbl)
                          }
                          frame "Timetrace" {
                            n4619 = local read "srateAODOtt"() -> (w1628:dbl)
                          }
                        }
                        n4620 = call "matlabwfexistsdialogue.vi"("Matlab waveform path"=w1624) -> ("mtalab waveform path out"=w1623:path)
                        n4621 = call "replace AO matlab param.vi"("Sampling frequency (Hz)"=w1621, "matlab wave file"=w1623, "index of AO wave"=w1626, "padding value"=w1625) -> ()  [unwired: 7 in]
                      }
                    }
                  }
                  frame #3 {
                    n4622 = case shown="True" w1629 {
                      tunnel: w1630 -> [_ w1637]
                      frame False {
                      }
                      frame True {
                        n4623 = local read "Meastab"() -> (w1634:enum32{"X-Y Image", "Linescan", "Timetrace"})
                        n4624 = call "waveformparamsv2.vi"("command"="get") -> ("Params out"=w1640:T14)  [unwired: 4 in, 2 out]
                        n4625 = Unbundle By Name(w1640) -> ("AO parameters"=w1639:T15)
                        n4626 = case shown="\"Timetrace\"" w1634 {
                          tunnel: [w1654 w1655] -> w1633
                          frame "X-Y Image", Default {
                            n4627 = local read "Sampling rate"() -> (w1654:dbl)
                          }
                          frame "Timetrace" {
                            n4628 = local read "srateAODOtt"() -> (w1655:dbl)
                          }
                        }
                        n4629 = Index Array(array=w1639, index=w1637) -> (element=w1638:T16)
                        n4630 = call "waveformsAObuffer.vi"("command"="get") -> ("AO wf out"=w1644:waveform(dbl)[])  [unwired: 1 in]
                        n4631 = call "matlabAOwffromparam.vi"("Cluster"=w1638) -> ("Waveform"=w1642:waveform(dbl))  [unwired: 1 out]
                        n4632 = property on="refwf" class="Ring (strict)"() -> ("RingText.Text"=w1645:string)  [unwired: 2 in, 2 out]
                        n4633 = Replace Array Subset(array=w1644, new element=w1642, index=w1637) -> (w1643:waveform(dbl)[])
                        n4634 = call "waveformsDObuffer.vi"("command"="get") -> ("DO wf out"=w1650:digitalwaveform[])  [unwired: 1 in]
                        n4635 = call "correctwaveformsizetemp.vi"("new sampling frequency (Hz)"=w1633, "start"=FALSE, "reference waveforms to"=w1645, "Analog waveforms in"=w1643, "stop"=FALSE, "Digital waveforms in"=w1650) -> ("analog wf out"=w1648:waveform(dbl)[], "Digital wf out"=w1646:digitalwaveform[], "measpoints"=w1635:i32)
                        n4636 = local read "wavdet"() -> (w1636:bool)
                        n4637 = local write "Analog Lines Plot"(w1648) -> ()
                        n4638 = call "GetNumCamFramesv2.vi"("Digital Waveform Graph"=w1646) -> ("Numeric"=w1647:i32)  [unwired: 10 in]
                        n4639 = local write "Digital Lines Plot"(w1646) -> ()
                        n4640 = call "waveformsAObuffer.vi"("AO wf in"=w1648, "command"="set") -> ()  [unwired: 1 out]
                        n4641 = call "waveformsDObuffer.vi"("DO wf in"=w1646, "command"="set") -> ()  [unwired: 1 out]
                        n4642 = local write "Total Camera Frames"(w1647) -> ()
                        n4643 = case shown="True" w1636 {
                          tunnel: w1635 -> [_ w1656]
                          frame False {
                          }
                          frame True {
                            n4644 = local write "# of frames"(w1656) -> ()
                          }
                        }
                      }
                    }
                  }
                  frame #4 {
                    w1658 = FALSE ("addAO")
                    n4645 = local read "finite samples"() -> (w1659:bool)
                    n4646 = local read "continuous"() -> (w1660:bool)
                    n4647 = local read "wavdet"() -> (w1661:bool)
                    n4648 = property on="Load Matlab Waveform" class="Bool (strict)"("Val(Sgnl)"=w1658) -> ()  [unwired: 2 in, 2 out]
                    n4649 = local write "changeAOmatlab"(w1658) -> ()
                    n4650 = local write "not loadedml"(FALSE ("not loadedml")) -> ()
                    n4651 = call "2pparameters.vi"("command"="get") -> ("params out"=w1664:T10)  [unwired: 1 in]
                    n4652 = Bundle By Name(cluster=w1664, "finite"=w1659, "cont"=w1660, "wavdet"=w1661) -> (w1662:T10)
                    n4653 = call "2pparameters.vi"("Params in"=w1662, "command"="set") -> ()  [unwired: 1 out]
                  }
                }
              }
            }
          }
          event "Load Matlab Waveform DO": Value Change {
            n4654 = event-data() -> ("NewVal"=w1666:bool)  [unwired: 1 in, 5 out]
            n4655 = case shown="True" w1666 {
              frame False {
              }
              frame True {
                n4656 = stacked-sequence {
                  seq-local: [_ _ w1774 _ _] -> [_ _ _ w1789 _]
                  seq-local: [_ _ w1773 _ _] -> [_ _ _ w1788 _]
                  frame #0 {
                    n4657 = local read "Measurement"() -> (w1668:T4)
                    n4658 = case shown="\"X-Y-t movie\", Default" w1668 {
                      frame "X-Y-t movie", Default {
                        n4659 = local read "avpp"() -> (w1689:i32)
                        n4660 = local read "Angle ref"() -> (w1688:dbl)
                        n4661 = local read "ROI Type"() -> (w1687:u16)
                        n4662 = local read "xpixels ref"() -> (w1684:i32)
                        n4663 = local read "Vx-min ref"() -> (w1683:dbl)
                        n4664 = local read "Vx-max ref"() -> (w1682:dbl)
                        n4665 = local read "ypixels ref"() -> (w1680:i32)
                        n4666 = local read "Vy-min ref"() -> (w1681:dbl)
                        n4667 = local read "Vy-max ref"() -> (w1677:dbl)
                        n4668 = local read "Sampling rate"() -> (w1671:dbl)
                        n4669 = local read "finite samples"() -> (w1672:bool)
                        n4670 = local read "continuous"() -> (w1675:bool)
                        n4671 = local read "wavdet"() -> (w1676:bool)
                        n4672 = local read "# of frames"() -> (w1674:i32)
                        n4673 = local read "maxbufferAI"() -> (w1673:i32)
                        n4674 = local read "Override AI buffer"() -> (w1669:bool)
                        n4675 = call "2pparameters.vi"("command"="get") -> ("params out"=w1686:T10)  [unwired: 1 in]
                        n4676 = Bundle By Name(cluster=w1686, "type"="X-Y-t movie", "avpp"=w1689, "Angle Img"=w1688, "Xpixels Img"=w1684, "Vx-min Img"=w1683, "VX-max Img"=w1682, "Ypixels Img"=w1680, "Vy-min Img"=w1681, "Vy-max Img"=w1677, "srate"=w1671, "srate Img"=w1671, "finite"=w1672, "cont"=w1675, "wavdet"=w1676, "measpoints"=w1674, "maxbufferAI"=w1673, "Drawing Mode"=w1687, "Vz-reset"=0.0, "AIoverride"=w1669) -> (w1678:T10)
                        n4677 = call "2pparameters.vi"("Params in"=w1678, "command"="set") -> ()  [unwired: 1 out]
                      }
                      frame "X-Y-Z stack" {
                        n4678 = call "2pparameters.vi"("command"="get") -> ("params out"=w1693:T10)  [unwired: 1 in]
                        n4679 = Bundle By Name(cluster=w1693, "type"="X-Y-Z stack") -> (w1691:T10)
                        n4680 = call "2pparameters.vi"("Params in"=w1691, "command"="set") -> ()  [unwired: 1 out]
                      }
                      frame "Lifetime (scan)" {
                        n4681 = call "2pparameters.vi"("command"="get") -> ("params out"=w1698:T10)  [unwired: 1 in]
                        n4682 = Bundle By Name(cluster=w1698, "type"="Lifetime (scan)") -> (w1696:T10)
                        n4683 = call "2pparameters.vi"("Params in"=w1696, "command"="set") -> ()  [unwired: 1 out]
                      }
                      frame "Lifetime (contour)" {
                        n4684 = local read "Vy-min draw"() -> (w1708:dbl)
                        n4685 = local read "Vy-max draw"() -> (w1707:dbl)
                        n4686 = local read "Vx-min draw"() -> (w1710:dbl)
                        n4687 = local read "Vx-max draw"() -> (w1709:dbl)
                        n4688 = local read "xpixels ref"() -> (w1706:i32)
                        n4689 = local read "ypixels ref"() -> (w1705:i32)
                        n4690 = local read "ROI Type"() -> (w1704:u16)
                        n4691 = local read "srateAODOtt"() -> (w1715:dbl)
                        n4692 = local read "# of frames"() -> (w1720:i32)
                        n4693 = local read "refreshtime"() -> (w1712:dbl)
                        n4694 = local read "Pel"() -> (w1703:dbl)
                        n4695 = local read "bin"() -> (w1718:dbl)
                        n4696 = local read "Override AI buffer"() -> (w1701:bool)
                        n4697 = local read "finite samples"() -> (w1727:bool)
                        n4698 = local read "srateAODOtt"() -> (w1714:dbl)
                        n4699 = local read "srateAODOtt"() -> (w1721:dbl)
                        n4700 = local read "continuous"() -> (w1726:bool)
                        n4701 = local read "Angle ref"() -> (w1711:dbl)
                        n4702 = local read "wavdet"() -> (w1728:bool)
                        n4703 = local read "Vx-ref"() -> (w1723:dbl)
                        n4704 = local read "Vy-ref"() -> (w1725:dbl)
                        n4705 = local read "avpp"() -> (w1724:i32)
                        n4706 = call "tt_timeandsamples.vi"("bin"=w1718, "refreshtime"=w1712, "srateAODOtt"=w1715, "tot#ofsamples"=w1720) -> ("refreshrate"=w1716:dbl, "refreshbuffer"=w1717:i32, "timetracecycles"=w1722:i32)  [unwired: 5 in]
                        n4707 = local read "bin"() -> (w1719:dbl)
                        n4708 = call "2pparameters.vi"("command"="get") -> ("params out"=w1731:T10)  [unwired: 1 in]
                        n4709 = Bundle By Name(cluster=w1731, "Drawing Mode"=w1704, "measpoints"=w1720, "tt_cycles"=w1722, "refreshbuffer"=w1717, "refreshrate"=w1716, "Vx-ref"=w1723, "Vy-ref"=w1725, "srate"=w1714, "finite"=w1727, "cont"=w1726, "wavdet"=w1728, "avpp"=w1724, "srateAODO"=w1721, "bufferAI"=w1717, "bin"=w1719, "Angle Img"=w1711, "Vxminref"=w1710, "Vxmaxref"=w1709, "Vyminref"=w1708, "Vymaxref"=w1707, "Xpixels Img"=w1706, "Ypixels Img"=w1705, "Pel"=w1703, "Vz-reset"=0.0, "AIoverride"=w1701, "type"="Lifetime (contour)") -> (w1729:T10)
                        n4710 = Reciprocal(x=w1716) -> (1/x=w1713:dbl)
                        n4711 = local write "refreshtime"(w1713) -> ()
                        n4712 = call "2pparameters.vi"("Params in"=w1729, "command"="set") -> ()  [unwired: 1 out]
                      }
                      frame "X-Y-Z-t movie" {
                      }
                      frame "linescan" {
                      }
                      frame "Timetrace" {
                        n4713 = local read "Vy-min draw"() -> (w1741:dbl)
                        n4714 = local read "Vy-max draw"() -> (w1740:dbl)
                        n4715 = local read "Vx-min draw"() -> (w1743:dbl)
                        n4716 = local read "Vx-max draw"() -> (w1742:dbl)
                        n4717 = local read "xpixels ref"() -> (w1739:i32)
                        n4718 = local read "ypixels ref"() -> (w1738:i32)
                        n4719 = local read "ROI Type"() -> (w1737:u16)
                        n4720 = local read "srateAODOtt"() -> (w1748:dbl)
                        n4721 = local read "# of frames"() -> (w1753:i32)
                        n4722 = local read "refreshtime"() -> (w1745:dbl)
                        n4723 = local read "Pel"() -> (w1736:dbl)
                        n4724 = local read "bin"() -> (w1751:dbl)
                        n4725 = local read "Override AI buffer"() -> (w1734:bool)
                        n4726 = local read "finite samples"() -> (w1760:bool)
                        n4727 = local read "srateAODOtt"() -> (w1747:dbl)
                        n4728 = local read "srateAODOtt"() -> (w1754:dbl)
                        n4729 = local read "continuous"() -> (w1759:bool)
                        n4730 = local read "Angle ref"() -> (w1744:dbl)
                        n4731 = local read "wavdet"() -> (w1761:bool)
                        n4732 = local read "Vx-ref"() -> (w1756:dbl)
                        n4733 = local read "Vy-ref"() -> (w1758:dbl)
                        n4734 = local read "avpp"() -> (w1757:i32)
                        n4735 = call "tt_timeandsamples.vi"("bin"=w1751, "refreshtime"=w1745, "srateAODOtt"=w1748, "tot#ofsamples"=w1753) -> ("refreshrate"=w1749:dbl, "refreshbuffer"=w1750:i32, "timetracecycles"=w1755:i32)  [unwired: 5 in]
                        n4736 = local read "bin"() -> (w1752:dbl)
                        n4737 = call "2pparameters.vi"("command"="get") -> ("params out"=w1764:T10)  [unwired: 1 in]
                        n4738 = Bundle By Name(cluster=w1764, "Drawing Mode"=w1737, "measpoints"=w1753, "tt_cycles"=w1755, "refreshbuffer"=w1750, "refreshrate"=w1749, "Vx-ref"=w1756, "Vy-ref"=w1758, "srate"=w1747, "finite"=w1760, "cont"=w1759, "wavdet"=w1761, "avpp"=w1757, "srateAODO"=w1754, "bufferAI"=w1750, "bin"=w1752, "Angle Img"=w1744, "Vxminref"=w1743, "Vxmaxref"=w1742, "Vyminref"=w1741, "Vymaxref"=w1740, "Xpixels Img"=w1739, "Ypixels Img"=w1738, "Pel"=w1736, "Vz-reset"=0.0, "AIoverride"=w1734, "type"="Timetrace") -> (w1762:T10)
                        n4739 = Reciprocal(x=w1749) -> (1/x=w1746:dbl)
                        n4740 = local write "refreshtime"(w1746) -> ()
                        n4741 = call "2pparameters.vi"("Params in"=w1762, "command"="set") -> ()  [unwired: 1 out]
                      }
                      frame "Lifetime (point)" {
                      }
                    }
                    n4742 = local write "changeDOmatlab"(TRUE ("addAO")) -> ()
                  }
                  frame #1 {
                    w1767 = FALSE ("wavdet")
                    n4743 = call "2pparameters.vi"("command"="get") -> ("params out"=w1771:T10)  [unwired: 1 in]
                    n4744 = Bundle By Name(cluster=w1771, "finite"=w1767, "cont"=w1767, "wavdet"=TRUE) -> (w1768:T10)
                    n4745 = call "2pparameters.vi"("Params in"=w1768, "command"="set") -> ()  [unwired: 1 out]
                  }
                  frame #2 {
                    n4746 = local read "DO channels"() -> (w1776:u16)
                    n4747 = call "2pparameters.vi"("command"="get") -> ("params out"=w1778:T10)  [unwired: 1 in]
                    n4748 = Unbundle By Name(w1778) -> ("aDO"=w1777:u32[])
                    n4749 = Search 1D Array(1D array=w1777, element=w1776) -> (index of element=w1774:i32)  [unwired: 1 in]
                    n4750 = Greater?(x=w1774, y=-1) -> (0:w1773:bool)
                    n4751 = case shown="True" w1773 {
                      tunnel: w1774 -> [_ w1785]
                      frame False {
                      }
                      frame True {
                        n4752 = local read "Meastab"() -> (w1781:enum32{"X-Y Image", "Linescan", "Timetrace"})
                        n4753 = local read "Matlab waveform path DO"() -> (w1783:path)
                        n4754 = local read "Matlab padding value DO"() -> (w1784:dbl)
                        n4755 = case shown="\"Timetrace\"" w1781 {
                          tunnel: [w1786 w1787] -> w1780
                          frame "X-Y Image", Default {
                            n4756 = local read "Sampling rate"() -> (w1786:dbl)
                          }
                          frame "Timetrace" {
                            n4757 = local read "srateAODOtt"() -> (w1787:dbl)
                          }
                        }
                        n4758 = call "matlabwfexistsdialogue.vi"("Matlab waveform path"=w1783) -> ("mtalab waveform path out"=w1782:path)
                        n4759 = call "replace DO matlab param.vi"("Sampling frequency (Hz)"=w1780, "matlab wave number"=w1782, "index of DO wave"=w1785, "padding value"=w1784) -> ()  [unwired: 7 in]
                      }
                    }
                  }
                  frame #3 {
                    n4760 = case shown="True" w1788 {
                      tunnel: w1789 -> [_ w1798]
                      frame False {
                      }
                      frame True {
                        n4761 = local read "Meastab"() -> (w1793:enum32{"X-Y Image", "Linescan", "Timetrace"})
                        n4762 = call "waveformparamsv2.vi"("command"="get") -> ("Params out"=w1811:T14)  [unwired: 4 in, 2 out]
                        n4763 = Unbundle By Name(w1811) -> ("DO parameters"=w1810:T17)
                        n4764 = case shown="\"Timetrace\"" w1793 {
                          tunnel: [w1813 w1814] -> w1792
                          frame "X-Y Image", Default {
                            n4765 = local read "Sampling rate"() -> (w1813:dbl)
                          }
                          frame "Timetrace" {
                            n4766 = local read "srateAODOtt"() -> (w1814:dbl)
                          }
                        }
                        n4767 = Index Array(array=w1810, index=w1798) -> (element=w1797:T18)
                        n4768 = call "waveformsDObuffer.vi"("command"="get") -> ("DO wf out"=w1808:digitalwaveform[])  [unwired: 1 in]
                        n4769 = property on="refwf" class="Ring (strict)"() -> ("RingText.Text"=w1800:string)  [unwired: 2 in, 2 out]
                        n4770 = call "matlabDOwffromparam.vi"("waveform params"=w1797) -> ("digital waveform"=w1796:digitalwaveform)
                        n4771 = Replace Array Subset(array=w1808, new element=w1796, index=w1798) -> (w1799:digitalwaveform[])
                        n4772 = call "waveformsAObuffer.vi"("command"="get") -> ("AO wf out"=w1807:waveform(dbl)[])  [unwired: 1 in]
                        n4773 = local read "wavdet"() -> (w1795:bool)
